vi "Console.vi"(6 "Buffer Size":i32=-1, 8 "Last Lines":refnum<vi>, 9 "Remote Console":refnum<vi>, 11 "Queue in":refnum<queue>) -> ()   [LabVIEW 2022 SP3]
uses:
  PythonCtrl.ctl
  Processors.ctl
panel:
  out "value":T1
  out "Console":string
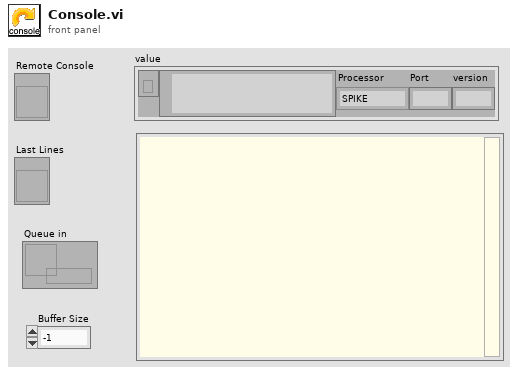
[diagram p1: front panel]
types:
  T1 = typedef "PythonCtrl.ctl" = cluster{"session":refnum<k35>, "PyPath":path, "Processor":T2, "Port":string, "version":string}
  T2 = typedef "Processors.ctl" = enum16{"SPIKE", "Pi", "Pi_ssh", "OpenMV", "Dunio"}
  T3 = enum8{"Enabled", "Disabled", "Disabled and Grayed Out"}
  T4 = typedef "eventvkey.ctl" = enum16{"ASCII", "Enter", "Return", "Shift", "Ctrl", "Alt", "Cmd", "Opt", "Caps", "NumLock", "Clear", "Break", "Up", "Down", "Left", "Right", "Insert", "Delete", "Home", "End", "PageUp", "PageDown", "Escape", "Help", "Pause", "ScrollLock", "F1", "F2", "F3", "F4", "F5", "F6", "F7", "F8", "F9", "F10", "F11", "F12", "F13", "F14", "F15", "F16", "F17", "F18", "F19", "F20", "F21", "F22", "F23", "F24", "Play", "VolumeUp", "VolumeDown", "Mute", "Two Byte Char"}
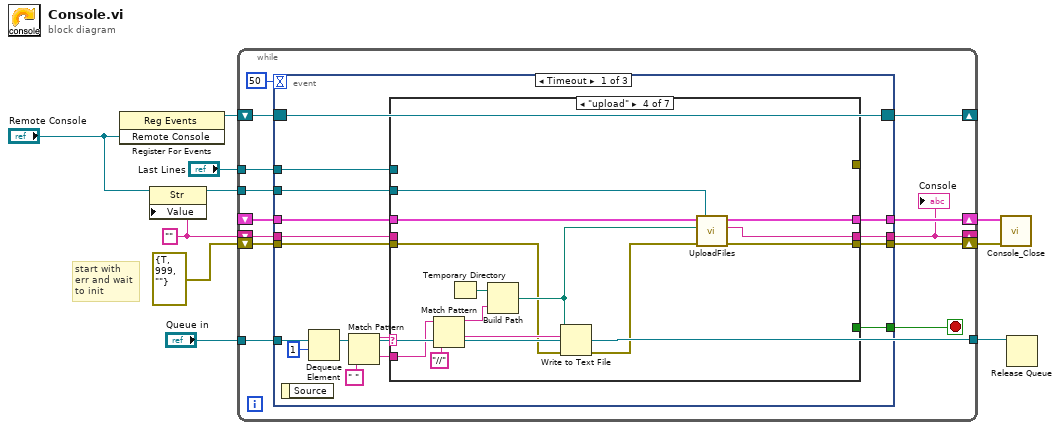
[diagram p0: block diagram]
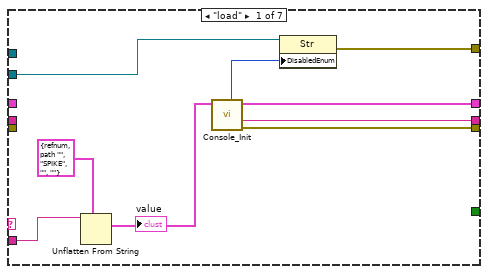
[diagram p2: hidden frame]
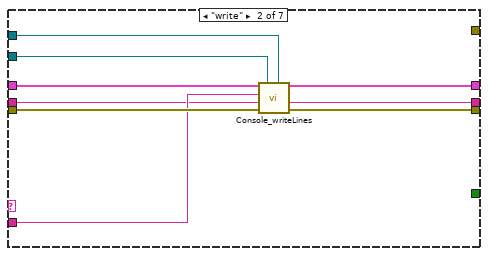
[diagram p3: hidden frame]
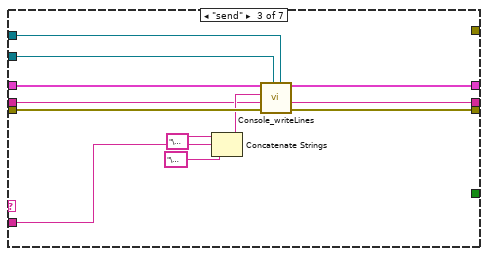
[diagram p4: hidden frame]
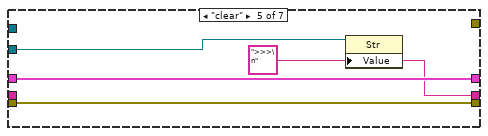
[diagram p5: hidden frame]
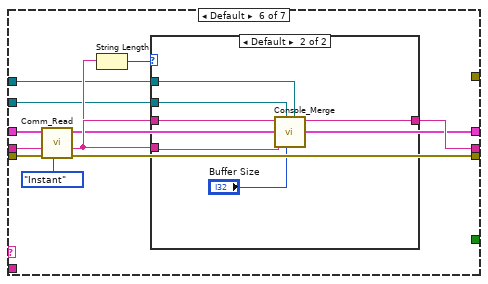
[diagram p6: hidden frame]
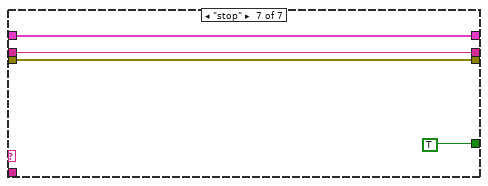
[diagram p8: hidden frame]
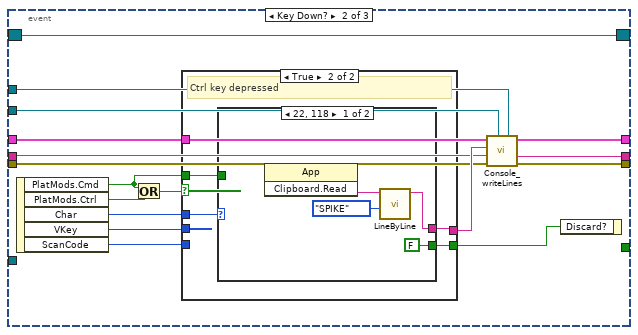
[diagram p9: hidden frame]
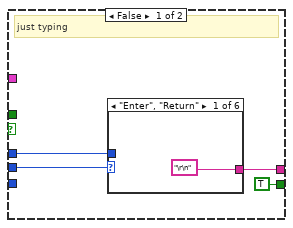
[diagram p10: hidden frame]
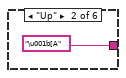
[diagram p11: hidden frame]
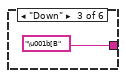
[diagram p12: hidden frame]
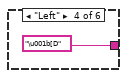
[diagram p13: hidden frame]
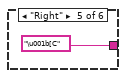
[diagram p14: hidden frame]
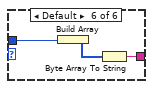
[diagram p15: hidden frame]
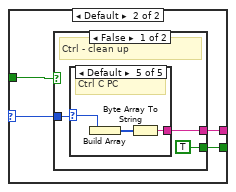
[diagram p16: hidden frame]
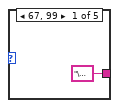
[diagram p17: hidden frame]
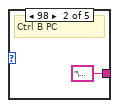
[diagram p18: hidden frame]
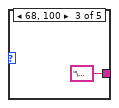
[diagram p19: hidden frame]
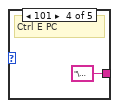
[diagram p20: hidden frame]
diagram:
  w1 = "" ("Console Out")
  # "start with\nerr and wait\nto init"
  n1 = register-events("Remote Console") -> (reference out=w9:refnum<event-registration>)  [unwired: 2 in, 1 out]
  n2 = property class="Str"(reference="Remote Console", "Value"=w1) -> ()  [unwired: 1 in, 2 out]
  n3 = while {
    shift-right: [w10] -> _
    shift-left: w1 -> [w22]
    tunnel: "Remote Console" -> [w18]
    shift-right: [w17] -> _
    shift-left: w9 -> [w19]
    tunnel: "Queue in" -> [w16]
    tunnel: [w16] -> w8
    shift-right: [w15] -> w5
    shift-left: _ -> [w14]
    tunnel: "Last Lines" -> [w11]
    shift-right: [w12] -> w6
    shift-left: errorcluster {"status"=TRUE, "code"=999, "source"=""} ("error out") -> [w13]
    stop <- w20 stop-if-true
    n4 = event shown="[0] Timeout" {
      selector: w19 -> [w32 w114 w163]
      dyn-events: [w32 w114 w163] -> w17
      timeout: u32 50 ("milliseconds to wait") -> [_ _ _]
      tunnel: w13 -> [w38 w110 w162]
      tunnel: w14 -> [w37 w113 w157]
      tunnel: w22 -> [w36 w106 w161]
      tunnel: [w35 w111 w162] -> w12
      tunnel: [w31 _ _] -> w20
      tunnel: [w34 w107 w161] -> w10
      tunnel: w18 -> [w33 w109 w158]
      tunnel: w16 -> [w28 _ _]
      tunnel: [w24 w113 w157] -> w15
      tunnel: w11 -> [w23 w108 _]
      event Timeout {
        n5 = event-data() -> ()  [unwired: 1 in, 1 out]
        n6 = Dequeue Element(queue=w28, timeout in ms (-1)=1) -> (element=w29:string)  [unwired: 1 in, 3 out]
        n7 = Match Pattern(string=w29, regular expression=" ") -> (before substring=w27:string, after substring=w26:string)  [unwired: 1 in, 2 out]
        n8 = case shown="\"upload\"" w27 {
          tunnel: w38 -> [_ w55 w63 w67 w82 w93 w103]
          tunnel: w37 -> [_ w52 w61 w76 w83 w85 w101]
          tunnel: w36 -> [_ w48 w56 _ _ w91 w102]
          tunnel: [w47 w54 w62 w78 w82 w90 w103] -> w35
          tunnel: [w43 w49 w57 w77 w80 w89 w102] -> w34
          tunnel: w33 -> [w46 w51 w59 w79 w81 w86 _]
          tunnel: [_ _ _ _ _ _ TRUE] -> w31
          tunnel: w26 -> [w41 w53 w64 w74 _ _ _]
          tunnel: [w42 w52 w61 w73 w83 w85 w101] -> w24
          tunnel: [w45 _ _ _ _ _ _] -> _
          tunnel: w23 -> [_ w50 w58 _ _ w84 _]
          frame "load" {
            n9 = Unflatten From String(type=T1 {"session"=refnum, "PyPath"=path "", "Processor"=enum."SPIKE", "Port"="", "version"=""} ("Python"), binary string=w41) -> (value=w39:T1)  [unwired: 3 in, 2 out]
            "value" <- w39
            n10 = call "Console_Init.vi"("Python"=w39) -> ("error out"=w47:errorcluster, "Console"=w43:string, "Python out"=w42:T1, "Disabled"=w44:T3)  [unwired: 7 in]
            n11 = property on="Property Node" class="Str"(reference=w46, "DisabledEnum"=w44) -> (error out=w45:errorcluster)  [unwired: 1 in, 1 out]
          }
          frame "write" {
            n12 = call "Console_writeLines.vi"("New Lines"=w50, "Console"=w51, "error in (no error)"=w55, "Console In"=w48, "code"=w53, "Python in"=w52) -> ("error out"=w54:errorcluster, "Console Out"=w49:string)  [unwired: 4 in]
          }
          frame "send" {
            n13 = Concatenate Strings("\u0005" ("queue"), w64, "\u0004" ("queue")) -> (w60:string)
            n14 = call "Console_writeLines.vi"("New Lines"=w58, "Console"=w59, "error in (no error)"=w63, "Console In"=w56, "code"=w60, "Python in"=w61) -> ("error out"=w62:errorcluster, "Console Out"=w57:string)  [unwired: 4 in]
          }
          frame "upload" {
            n15 = Match Pattern(string=w74, regular expression="//") -> (before substring=w70:string, after substring=w72:string)  [unwired: 1 in, 2 out]
            n16 = Temporary Directory() -> (w71:path)
            n17 = Build Path(base path=w71, name or relative path=w70) -> (appended path=w69:path)
            n18 = Write to Text File(file (use dialog)=w69, text=w72, error in=w67) -> (error out=w68:errorcluster)  [unwired: 1 in, 2 out]
            n19 = call "UploadFiles.vi"("error in (no error)"=w68, "Python in"=w76, "path"=w69, "Console"=w79) -> ("error out"=w78:errorcluster, "Console out"=w77:string, "Python out"=w73:T1)  [unwired: 5 in]
          }
          frame "clear" {
            w80 = ">>>\n" ("Console Out")
            n20 = property class="Str"(reference=w81, "Value"=w80) -> ()  [unwired: 1 in, 2 out]
          }
          frame Default {
            n21 = call "Comm_Read.vi"("Task"=enum16{"Instant", "All", "AllFast", "Params"}."Instant", "error in (no error)"=w93, "Python"=w85) -> ("error out"=w90:errorcluster, "Text read"=w88:string)  [unwired: 7 in]
            n22 = String Length(string=w88) -> (length=w87:i32)
            n23 = case shown="Default" w87 {
              tunnel: w88 -> [_ w97]
              tunnel: w91 -> [w94 w98]
              tunnel: [w94 w100] -> w89
              tunnel: w86 -> [_ w99]
              tunnel: w84 -> [_ w95]
              frame 0 {
              }
              frame Default {
                n24 = call "Console_Merge.vi"("New Lines"=w95, "Buffer Size"="Buffer Size", "Console"=w99, "Text read"=w97, "Console In"=w98) -> ("Console Out"=w100:string)  [unwired: 6 in]
              }
            }
          }
          frame "stop" {
          }
        }
      }
      event Key Down? {
        n25 = event-data() -> ("PlatMods.Cmd"=w115:bool, "PlatMods.Ctrl"=w118:bool, "Char"=w119:i16, "VKey"=w120:T4, "ScanCode"=w105:i16)  [unwired: 1 in]
        n26 = Or(x=w115, y=w118) -> (x .or. y?=w117:bool)
        n27 = case shown="True" w117 {
          tunnel: [w124 w136] -> w112
          tunnel: w120 -> [w123 _]
          tunnel: w119 -> [w122 w133]
          tunnel: [TRUE ("Discard?") w135] -> w116
          tunnel: w115 -> [_ w134]
          tunnel: w113 -> [_ _]
          tunnel: w105 -> [_ _]
          frame False {
            # "just typing"
            n28 = case shown="\"Enter\", \"Return\"" w123 {
              tunnel: w122 -> [_ _ _ _ _ w132]
              tunnel: ["\r\n" ("replace string (\"\")") "\u001b[A" ("replace string (\"\")") "\u001b[B" ("replace string (\"\")") "\u001b[D" ("replace string (\"\")") "\u001b[C" ("replace string (\"\")") w131] -> w124
              frame "Enter", "Return" {
              }
              frame "Up" {
              }
              frame "Down" {
              }
              frame "Left" {
              }
              frame "Right" {
              }
              frame Default {
                n29 = Build Array(w132) -> (w130:i16[])
                n30 = Byte Array To String(unsigned byte array=w130) -> (string=w131:string)
              }
            }
          }
          frame True {
            # "Ctrl key depressed"
            n31 = case shown="22, 118" w133 {
              selector: w133 -> [_ w141]
              tunnel: [w137 w144] -> w136
              tunnel: [FALSE ("Discard?") w143] -> w135
              tunnel: w134 -> [_ w142]
              frame 22, 118 {
                n32 = invoke class="App" method="Clipboard.Read"() -> ("Read Clipbrd"=w139:string)  [unwired: 3 in, 2 out]
                n33 = call "LineByLine.vi"("Processor"=enum16{"SPIKE", "Pi"}."SPIKE", "Python Code"=w139) -> ("result string"=w137:string)  [unwired: 9 in]
              }
              frame Default {
                n34 = case shown="False" w142 {
                  tunnel: [w147 "" ("string")] -> w144
                  tunnel: w141 -> [w145 _]
                  tunnel: [TRUE ("Discard?") FALSE ("Discard?")] -> w143
                  frame False {
                    # "Ctrl - clean up"
                    n35 = case shown="Default" w145 {
                      selector: w145 -> [_ _ _ _ w152]
                      tunnel: ["\u0003" ("string") "\u0002" ("string") "\u0004" ("string") "\u0005" ("string") w153] -> w147
                      frame 67, 99 {
                      }
                      frame 98 {
                        # "Ctrl B PC"
                      }
                      frame 68, 100 {
                      }
                      frame 101 {
                        # "Ctrl E PC"
                      }
                      frame Default {
                        # "Ctrl C PC"
                        n36 = Build Array(w152) -> (w154:i16[])
                        n37 = Byte Array To String(unsigned byte array=w154) -> (string=w153:string)
                      }
                    }
                  }
                  frame True {
                    # "Cmd C/V use OS"
                  }
                }
              }
            }
          }
        }
        n38 = call "Console_writeLines.vi"("New Lines"=w108, "Console"=w109, "error in (no error)"=w110, "Console In"=w106, "code"=w112, "Python in"=w113) -> ("error out"=w111:errorcluster, "Console Out"=w107:string)  [unwired: 4 in]
        n39 = event-data("Discard?"=w116) -> ()  [unwired: 1 in, 1 out]
      }
      event Panel Resize {
        n40 = event-data() -> ()  [unwired: 1 in, 8 out]
        n41 = property on="Property Node" class="Str"(reference=w158, "Key Focus"=TRUE, "Text.Scroll Position"=u32 9999999) -> ()  [unwired: 1 in, 2 out]
      }
    }
    "Console" <- w10
  }
  n42 = call "Console_Close.vi"("error in (no error)"=w6, "Python in"=w5) -> ()  [unwired: 9 in, 1 out]
  n43 = Release Queue(queue=w8) -> ()  [unwired: 2 in, 3 out]
